vi "generateAnalyticalModel.vi"(8 "error in (no error)":errorcluster, 11 "Game in":refnum<class "Game.lvclass">) -> (0 "error out":errorcluster, 3 "Game out":refnum<class "Game.lvclass">)   [LabVIEW 2023, in "Game.lvclass"]
uses:
  Game.lvclass
  Controls/RobotModelTestState.ctl
  Robot_class/Robot.lvclass
  C:/Users/ebert/Desktop/roboime/SSL_AI/Object_class/Object.lvclass
  Communication_class/Paths/grSim Packet Command UDP Test Folder/grSim/grSim RobotReplacement.ctl
  Ally_class/Ally.lvclass
  C:/Users/ebert/Desktop/roboime/SSL_AI/Team_class/Team.lvclass
  <vilib>/Analysis/Matrix/Datatypes/RealMatrix.ctl
  Game.lvclass/Game.ctl
  Object_class/Object.lvclass/Object.ctl
  Robot_class/Robot.lvclass/Robot.ctl
  Team_class/Team.lvclass/Team.ctl
  Object_class/Write x.vi
  Robot_class/Write est_v_tang.vi
  Team_class/Write RobotRef.vi
  Write AllyRef.vi
  Team_class/Read RobotRef.vi
  Robot_class/Read v_tang.vi
  Read AllyRef.vi
  <vilib>/Analysis/Matrix/NI_Matrix.lvlib
panel:
  out "State 2":T1 {"progress" scale=0.0..100.0}
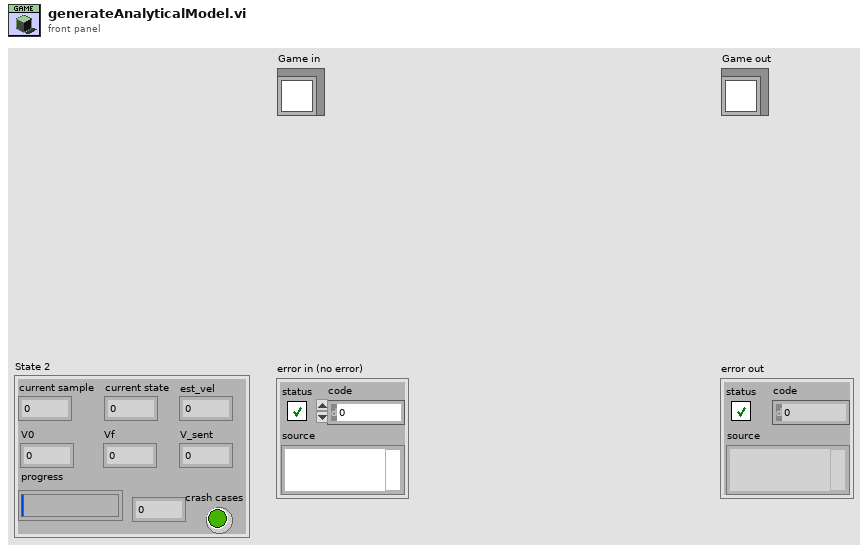
[diagram p1: front panel]
types:
  T1 = typedef "RobotModelTestState.ctl" = cluster{"current sample":i32, "V0":dbl, "Vf":dbl, "progress":dbl, "current state":i32, "est_vel":dbl, "V_sent":dbl, "crash cases":bool}
  T2 = typedef "grSim RobotReplacement.ctl" = cluster{"x":dbl, "y":dbl, "dir(degree)":dbl, "yellowteam":bool, "id":u32}
  T3 = typedef "NI_Matrix.lvlib/RealMatrix.ctl" = dbl[][]
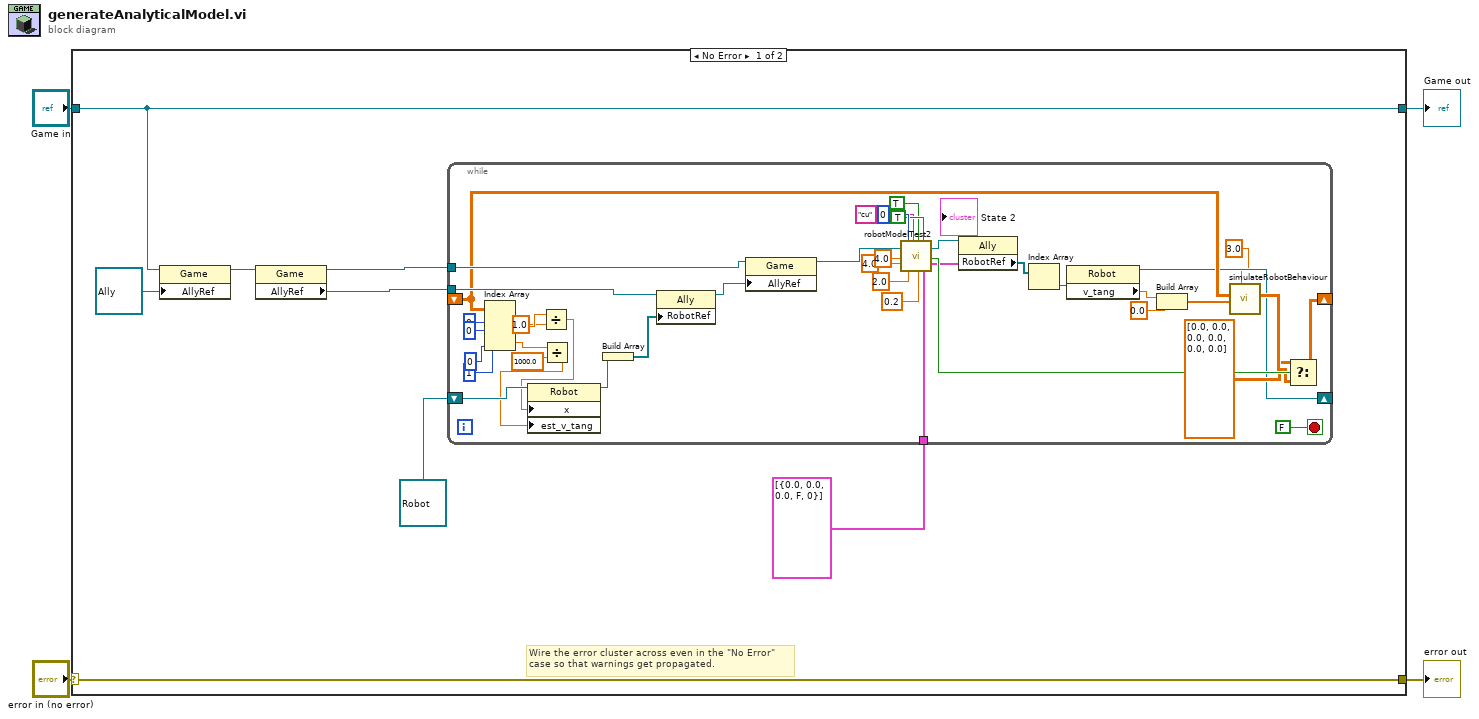
[diagram p0: block diagram]
diagram:
  n1 = case shown="No Error" "error in (no error)" {
    selector: "error in (no error)" -> [w12 w55]
    tunnel: [w12 w55] -> w3
    tunnel: [w7 w54] -> w1
    tunnel: "Game in" -> [w7 w54]
    frame No Error {
      # "Wire the error cluster across even in the \"No Error\"\ncase so that warnings get propagated."
      n2 = property class="Game"(reference=w7, "AllyRef"=refnum<class "Ally.lvclass"> refnum) -> (reference out=w5:refnum<class "Game.lvclass">)  [unwired: 1 in, 1 out]
      n3 = property class="Game"(reference=w5) -> (reference out=w9:refnum<class "Game.lvclass">, "AllyRef"=w11:refnum<class "Ally.lvclass">)  [unwired: 1 in, 1 out]
      n4 = while {
        tunnel: w11 -> [w53]
        tunnel: w9 -> [w46]
        tunnel: T2[] [{"x"=0.0, "y"=0.0, "dir(degree)"=0.0, "yellowteam"=FALSE, "id"=0}] ("grSIM replacement.robots") -> [w37]
        shift-right: [w21] -> _
        shift-left: _ -> [w25]
        shift-right: [w18] -> _
        shift-left: refnum<class "Robot.lvclass"> refnum ("element") -> [w31]
        stop <- FALSE stop-if-true
        n5 = Index Array(array=w25, index (row) #1=0 ("disabled index (row)"), index (col) #1=0 ("disabled index (col)"), index (row) #2=1 ("disabled index (row)"), index (col) #2=0 ("index (col)")) -> (element #1=w29:dbl, element #2=w28:dbl)
        n6 = Divide(x=w29, y=1.0) -> (x/y=w27:dbl)
        n7 = Divide(x=w28, y=1000.0) -> (x/y=w26:dbl)
        n8 = property class="Robot"(reference=w31, "x"=w27, "est_v_tang"=w26) -> (reference out=w30:refnum<class "Robot.lvclass">)  [unwired: 1 in, 1 out]
        n9 = Build Array(w30) -> (w47:refnum<class "Robot.lvclass">[])
        n10 = property class="Ally"(reference=w53, "RobotRef"=w47) -> (reference out=w45:refnum<class "Ally.lvclass">)  [unwired: 1 in, 1 out]
        n11 = property class="Game"(reference=w46, "AllyRef"=w45) -> (reference out=w44:refnum<class "Game.lvclass">)  [unwired: 1 in, 1 out]
        n12 = call "robotModelTest2.vi"("Game in"=w44, "V_sent"=4.0, "V_sample"=4.0, "id"=0, "Samples"=2.0, "RobotModelFolder"="cu", "Start"=TRUE, "delta"=0.2, "replace active"=TRUE, "grSIM replacement.robots"=w37) -> ("TestTeam"=w43:refnum<class "Ally.lvclass">, "Replace"=w24:bool, "State"=→"State 2":T1)  [unwired: 5 in, 2 out]
        n13 = property class="Ally"(reference=w43) -> ("RobotRef"=w42:refnum<class "Robot.lvclass">[])  [unwired: 1 in, 2 out]
        n14 = Index Array(array=w42) -> (element=w41:refnum<class "Robot.lvclass">)  [unwired: 1 in]
        n15 = property class="Robot"(reference=w41) -> (reference out=w18:refnum<class "Robot.lvclass">, "v_tang"=w40:dbl)  [unwired: 1 in, 1 out]
        n16 = Build Array(w40, 0.0 ("element")) -> (w38:dbl[])
        n17 = call "simulateRobotBehaviour.vi"("max_accel"=3.0, "u_k"=w38, "x_k_k"=w25) -> ("x_k+1"=w23:T3)  [unwired: 6 in, 2 out]
        n18 = Select(t=T3 [[0.0], [0.0], [0.0], [0.0], [0.0], [0.0]], s=w24, f=w23) -> (s? t:f=w21:T3)
      }
    }
    frame Error {
    }
  }
  "error out" <- w3
  "Game out" <- w1
